vi "TCP-Receive (1D SGL).vi"(0 "connection ID":refnum<k5>, 9 "timeout (ms)":i32=5000, 11 "error in (no error)":errorcluster) -> (4 "connection ID out":refnum<k5>, 8 "Array":sgl[](array[numeric]), 15 "error out":errorcluster)   [LabVIEW 2020]
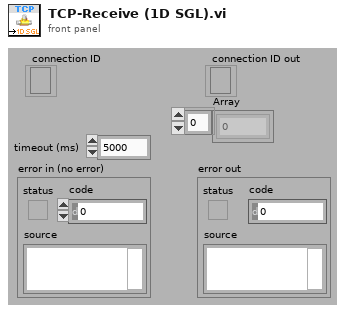
[diagram p1: front panel]
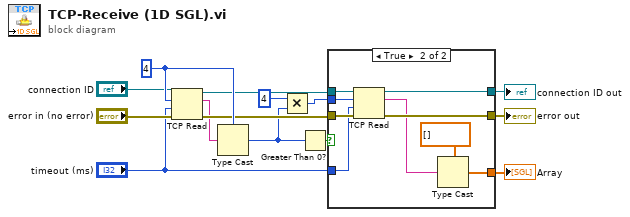
[diagram p0: block diagram]
diagram:
  w14 = 4
  n1 = TCP Read(connection ID="connection ID", bytes to read=w14, error in (no error)="error in (no error)", 9:"timeout (ms)") -> (connection ID out=w11:refnum<k5>, data out=w5:string, error out=w12:errorcluster)  [unwired: 1 in]
  n2 = Type Cast(type=w14, x=w5) -> (*(type *) &x=w2:i32)
  n3 = Multiply(x=4, y=w2) -> (x*y=w3:i32)
  n4 = Greater Than 0?(x=w2) -> (x > 0?=w9:bool)
  n5 = case shown="True" w9 {
    tunnel: [w16 w25] -> w8
    tunnel: w11 -> [w15 w24]
    tunnel: w12 -> [w16 w23]
    tunnel: w3 -> [_ w22]
    tunnel: [w15 w21] -> w10
    tunnel: "timeout (ms)" -> [_ w20]
    tunnel: [_ w17] -> w4
    frame False {
    }
    frame True {
      n6 = TCP Read(connection ID=w24, bytes to read=w22, error in (no error)=w23, 9:w20) -> (connection ID out=w21:refnum<k5>, data out=w19:string, error out=w25:errorcluster)  [unwired: 1 in]
      n7 = Type Cast(type=sgl[] [], x=w19) -> (*(type *) &x=w17:sgl[])
    }
  }
  "error out" <- w8
  "connection ID out" <- w10
  "Array" <- w4
